vi "Stop Core.vi"(10 "final error code":i32, 11 "Alpha UI in":refnum<class "Simulated Entry Console.lvclass">) -> (3 "Alpha UI out":refnum<class "Simulated Entry Console.lvclass">)   [LabVIEW 2012, in "Simulated Entry Console.lvlib" / "Simulated Entry Console.lvclass"]
doc: "(<B>Filename</B>: Actor Framework.lvlib:Actor.lvclass:Stop Core.vi)\n\nDefines what the actor does before it stops. Use the <B>final error code</B> input to determine whether the actor shut down in response to an error.\n\nBy default, this method does nothing. A descendant class may override it to define behavior, such as shutting down any processes the actor initiated in its override of the Actor Core method."
uses:
  Simulated Entry Console.lvclass
  Entry Console API/Entry Console API/Entry Console API.lvclass
  Simulated Entry Console.lvclass/Simulated Entry Console.ctl
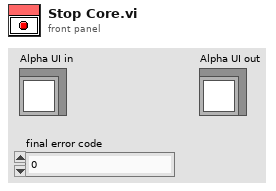
[diagram p1: front panel]
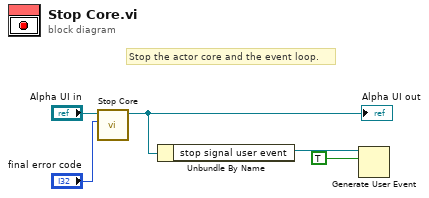
[diagram p0: block diagram]
diagram:
  # "Stop the actor core and the event loop."
  n1 = call-parent "Stop Core.vi"("final error code"="final error code", "Actor in"="Alpha UI in") -> ("Actor out"=w3:refnum<class "Simulated Entry Console.lvclass">)  [unwired: 9 in]
  "Alpha UI out" <- w3
  n2 = Unbundle By Name(w3) -> ("stop signal user event"=w2:refnum<user-event>)
  n3 = Generate User Event(user event=w2, event data cluster=TRUE ("event data")) -> ()  [unwired: 1 in, 2 out]
